vi "Autotune.vi"(1 "Adjust Tune":bool, 2 "Tune Vin":dbl, 3 "Pedestal Diff":dbl[](array[numeric])) -> (0 "Tune Vout":dbl)   [LabVIEW 2013]
uses:
  <vilib>/Analysis/NI_AALBase.lvlib
panel:
  # "Adjusts tuner voltage  for flat pedestal"
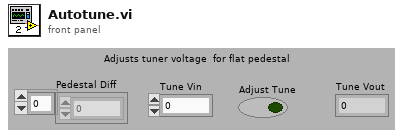
[diagram p1: front panel]
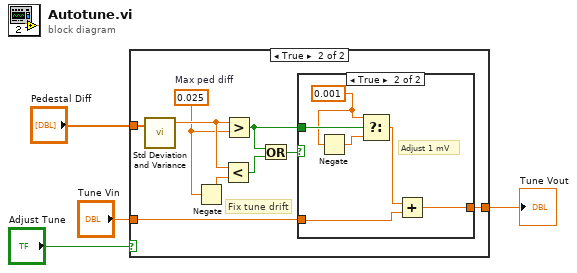
[diagram p0: block diagram]
diagram:
  n1 = case shown="True" "Adjust Tune" {
    tunnel: "Pedestal Diff" -> [_ w14]
    tunnel: "Tune Vin" -> [w5 w7]
    tunnel: [w5 w6] -> w4
    frame False {
    }
    frame True {
      w12 = 0.025  # Max ped diff
      # "Fix tune drift"
      n2 = call <vilib>:"Std Deviation and Variance.vi"("X"=w14) -> ("mean"=w13:dbl)  [unwired: 1 in, 2 out]
      n3 = Negate(x=w12) -> (-x=w11:dbl)
      n4 = Less?(x=w13, y=w11) -> (x < y?=w10:bool)
      n5 = Greater?(x=w13, y=w12) -> (0:w8:bool)
      n6 = Or(x=w8, y=w10) -> (x .or. y?=w9:bool)
      n7 = case shown="True" w9 {
        tunnel: w8 -> [_ w21]
        tunnel: w7 -> [w15 w17]
        tunnel: [w15 w16] -> w6
        frame False {
        }
        frame True {
          w19 = 0.001
          # "Adjust 1 mV"
          n8 = Negate(x=w19) -> (-x=w20:dbl)
          n9 = Select(t=w19, s=w21, f=w20) -> (s? t:f=w18:dbl)
          n10 = Add(x=w18, y=w17) -> (x+y=w16:dbl)
        }
      }
    }
  }
  "Tune Vout" <- w4
